vi "VIV_VIPM Post Uninstall Process.vi"(8 "Error In":errorcluster, 11 "PackageName":string) -> (0 "Error Out":errorcluster)   [LabVIEW 2018]
uses:
  <vilib>/Utility/file.llb/Read Delimited Spreadsheet (string).vi
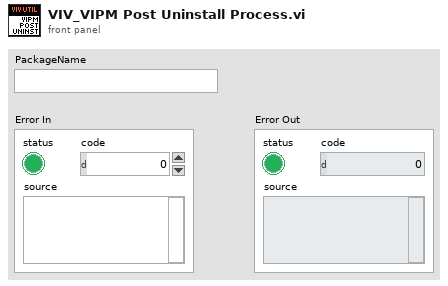
[diagram p1: front panel]
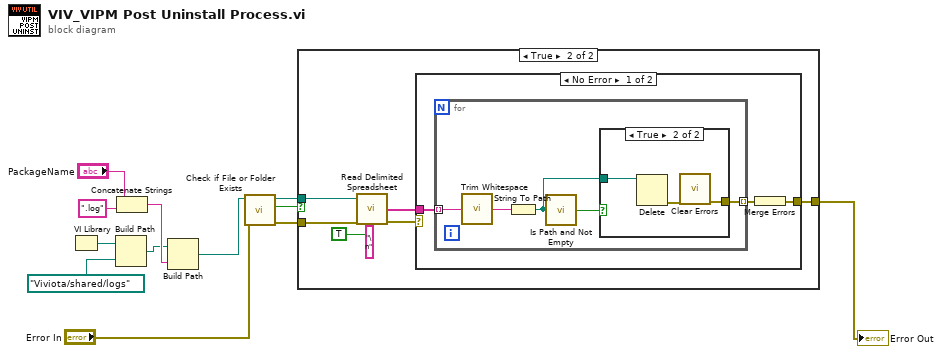
[diagram p0: block diagram]
diagram:
  n1 = VI Library() -> (path=w6:path)
  n2 = Build Path(base path=w6, name or relative path=path "Viviota/shared/logs") -> (appended path=w4:path)
  n3 = Concatenate Strings("PackageName", ".log" ("string")) -> (w11:string)
  n4 = Build Path(base path=w4, name or relative path=w11) -> (appended path=w7:path)
  n5 = call <vilib>:"Check if File or Folder Exists.vi"("error in (no error)"="Error In", "path"=w7) -> ("error out"=w8:errorcluster, "file or folder exists?"=w10:bool, "dup path"=w9:path)  [unwired: 7 in]
  n6 = case shown="True" w10 {
    tunnel: w9 -> [_ w20]
    tunnel: w8 -> [w13 w17]
    tunnel: [w13 w14] -> w1
    frame False {
    }
    frame True {
      n7 = call-poly <vilib>:"Read Delimited Spreadsheet.vi"("file path (dialog if empty)"=w20, "error in (no error)"=w17, "transpose? (F)"=TRUE, "delimiter (\\t)"="\n" ("delimiter (\\t)")) -> ("first row"=w18:string[], "error out"=w16:errorcluster)  [unwired: 6 in, 4 out]
      n8 = case shown="No Error" w16 {
        selector: w16 -> [_ w32]
        tunnel: w18 -> [w23 _]
        tunnel: [w21 w32] -> w14
        frame No Error {
          n9 = for {
            tunnel: w23 -> [w28] mode=indexing
            tunnel: [w24] -> w22 mode=indexing
            n10 = call <vilib>:"Trim Whitespace.vi"("string"=w28) -> ("trimmed string"=w27:string)  [unwired: 1 in]
            n11 = String To Path(string=w27) -> (path=w25:path)
            n12 = call <vilib>:"Is Path and Not Empty.vi"("path"=w25) -> ("Is Path and Not Empty?"=w26:bool)  [unwired: 4 in]
            n13 = case shown="True" w26 {
              tunnel: w25 -> [_ w31]
              tunnel: [_ w29] -> w24
              frame False {
              }
              frame True {
                n14 = Delete(path (use dialog)=w31) -> (error out=w30:errorcluster)  [unwired: 4 in, 2 out]
                n15 = call <vilib>:"Clear Errors.vi"("error in (no error)"=w30) -> ("error out"=w29:errorcluster)  [unwired: 5 in, 1 out]
              }
            }
          }
          n16 = Merge Errors(w22) -> (w21:errorcluster)
        }
        frame Error {
        }
      }
    }
  }
  "Error Out" <- w1
